vi "Read ATM.vi"(8 "error in (no error)":errorcluster, 11 "AlicatPressureController in":refnum<class "AlicatPressureController.lvclass">) -> (0 "error out":errorcluster, 3 "AlicatPressureController out":refnum<class "AlicatPressureController.lvclass">)   [LabVIEW 2020, in "AlicatPressureController.lvclass"]
uses:
  AlicatPressureController.lvclass
  OnOffTypeDef.ctl
  AlicatPressureController.lvclass/AlicatPressureController.ctl
panel:
  out ">Current ATM >":dbl
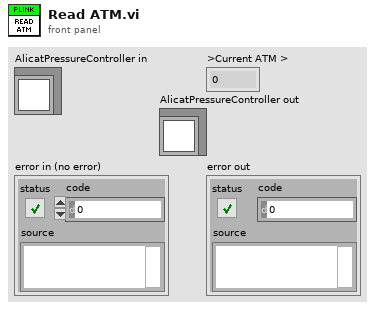
[diagram p1: front panel]
types:
  T1 = typedef "OnOffTypeDef.ctl" = enum16{"off", "on"}
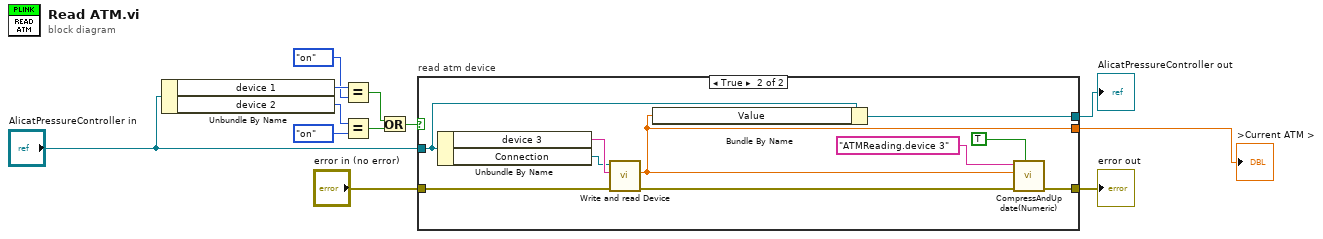
[diagram p0: block diagram]
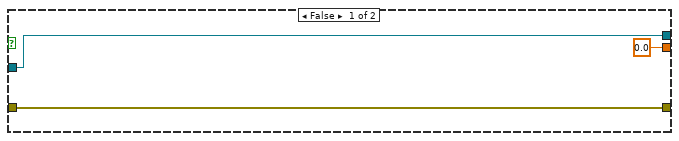
[diagram p2: hidden frame]
diagram:
  n1 = Unbundle By Name("AlicatPressureController in") -> ("device 1"=w10:T1, "device 2"=w6:T1)
  n2 = Equal?(x=w10, y=OnOffTypeDef."on" ("Settings.AtmReader.device 2")) -> (x = y?=w4:bool)
  n3 = Equal?(x=w6, y=OnOffTypeDef."on" ("Settings.AtmReader.device 2")) -> (x = y?=w5:bool)
  n4 = Or(x=w4, y=w5) -> (x .or. y?=w8:bool)
  n5 = case "read atm device" shown="True" w8 {
    tunnel: [0.0 ("pressure reading") w17] -> w12
    tunnel: "AlicatPressureController in" -> [w13 w18]
    tunnel: "error in (no error)" -> [w14 w23]
    tunnel: [w14 w19] -> w11
    tunnel: [w13 w16] -> w1
    frame False {
    }
    frame True {
      n6 = Unbundle By Name(w18) -> ("device 3"=w25:string, "Connection"=w24:refnum<visa-resource-name>)
      n7 = call "Write and read Device.vi"("error in (no error)"=w23, "device 1"=w25, "VISA Refnum in"=w24) -> ("error out"=w22:errorcluster, "pressure reading"=w17:dbl)  [unwired: 5 in, 2 out]
      n8 = Bundle By Name(cluster=w18, "Value"=w17) -> (w16:refnum<class "AlicatPressureController.lvclass">)
      n9 = call "CompressAndUpdate(Numeric).vi"("force CVT update (false)"=TRUE, "error in"=w22, "Numeric"=w17, "command or variable name"="ATMReading.device 3") -> ("error out"=w19:errorcluster)  [unwired: 7 in]
    }
  }
  ">Current ATM >" <- w12
  "error out" <- w11
  "AlicatPressureController out" <- w1
